vi "Delete Subordinate Object Queue.vi"(8 "error in (no error)":errorcluster, 9 "Name":string, 10 "Caller-To-Actor Enqueuer":refnum<class "Message Enqueuer.lvclass">, 11 "Template Module in":refnum<class "Template Module.lvclass">) -> (0 "error out":errorcluster, 3 "Template Module out":refnum<class "Template Module.lvclass">)   [LabVIEW 2019, in "Template Module.lvclass"]
uses:
  Template Module.lvclass
  <vilib>/ActorFramework/Message Enqueuer/Message Enqueuer.lvclass
  Template Module.lvclass/Template Module.ctl
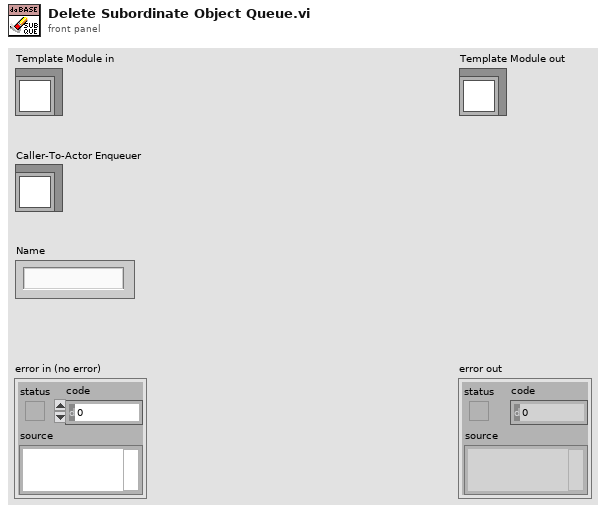
[diagram p1: front panel]
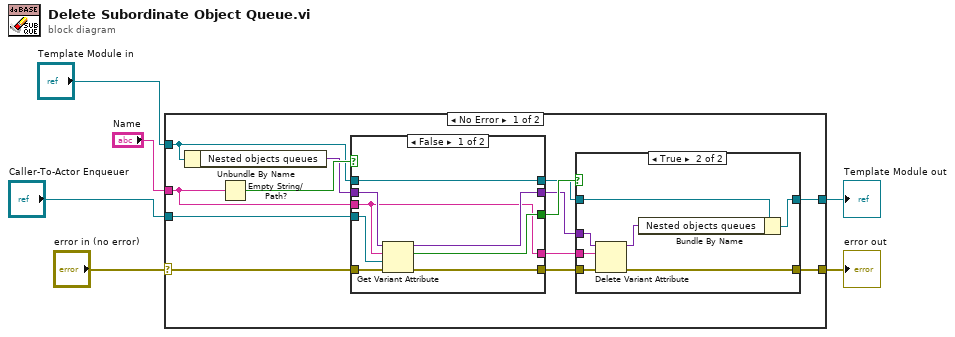
[diagram p0: block diagram]
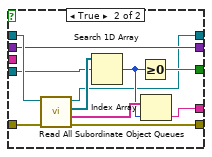
[diagram p3: hidden frame]
diagram:
  n1 = case shown="No Error" "error in (no error)" {
    selector: "error in (no error)" -> [w15 w49]
    tunnel: [w8 w49] -> w5
    tunnel: [w7 w48] -> w3
    tunnel: "Template Module in" -> [w14 w48]
    tunnel: "Name" -> [w17 _]
    tunnel: "Caller-To-Actor Enqueuer" -> [w16 _]
    frame No Error {
      n2 = Unbundle By Name(w14) -> ("Nested objects queues"=w18:variant)
      n3 = Empty String/Path?(string/path=w17) -> (empty?=w19:bool)
      n4 = case shown="False" w19 {
        tunnel: w18 -> [w36 w38]
        tunnel: w17 -> [w30 _]
        tunnel: w16 -> [w35 w44]
        tunnel: w15 -> [w34 w46]
        tunnel: [w33 w43] -> w13
        tunnel: [w32 w38] -> w12
        tunnel: [w31 w42] -> w10
        tunnel: w14 -> [w29 w47]
        tunnel: [w30 w39] -> w11
        tunnel: [w29 w37] -> w9
        frame False {
          n5 = Get Variant Attribute(Variant=w36, name=w30, default value (empty Variant)=w35, error in=w34) -> (duplicate Variant=w32:variant, found=w33:bool, error out=w31:errorcluster)  [unwired: 1 out]
        }
        frame True {
          n6 = call-dynamic "Read All Subordinate Object Queues.vi"("error in (no error)"=w46, "Measure Object in"=w47) -> ("error out"=w42:errorcluster, "Object names"=w41:string[], "Object enqueuers"=w45:refnum<class "Message Enqueuer.lvclass">[], "Measure Object out"=w37:refnum<class "Template Module.lvclass">)  [unwired: 6 in]
          n7 = Search 1D Array(1D array=w45, element=w44) -> (index of element=w40:i32)  [unwired: 1 in]
          n8 = Greater Or Equal To 0?(x=w40) -> (x >= 0?=w43:bool)
          n9 = Index Array(array=w41, index=w40) -> (element=w39:string)
        }
      }
      n10 = case shown="True" w13 {
        tunnel: w12 -> [_ w28]
        tunnel: w11 -> [_ w27]
        tunnel: w10 -> [w21 w26]
        tunnel: w9 -> [w20 w25]
        tunnel: [w21 w23] -> w8
        tunnel: [w20 w22] -> w7
        frame False {
        }
        frame True {
          n11 = Delete Variant Attribute(4:w26, 6:w27, 7:w28) -> (0:w23:errorcluster, 3:w24:variant)  [unwired: 1 out]
          n12 = Bundle By Name(cluster=w25, "Nested objects queues"=w24) -> (w22:refnum<class "Template Module.lvclass">)
        }
      }
    }
    frame Error {
    }
  }
  "error out" <- w5
  "Template Module out" <- w3
